vi "getControlMatrixDH.vi"(8 "error in (no error)":errorcluster, 11 "DataHandler in":refnum<class "DataHandler.lvclass">) -> (0 "error out":errorcluster, 1 "List of ColHads":string[](array[string]), 2 "ControlParameterArrayMatrix":string[][](array[string]), 3 "DataHandler out":refnum<class "DataHandler.lvclass">, 4 "Field Elements":string[](array[string]))   [LabVIEW 2017, in "DataHandler.lvclass"]
uses:
  DataHandler.lvclass
  DataHandler.lvclass/DataHandler.ctl
  <vilib>/drjdpowell/SQLite Library/SQL Connection/Execute SQL.vi
  <vilib>/drjdpowell/SQLite Library/SQLite.lvlib
  <vilib>/drjdpowell/SQLite Library/SQL Connection/Connection.lvclass
panel:
  in  "Control-Matrix":i32(listbox)=-1
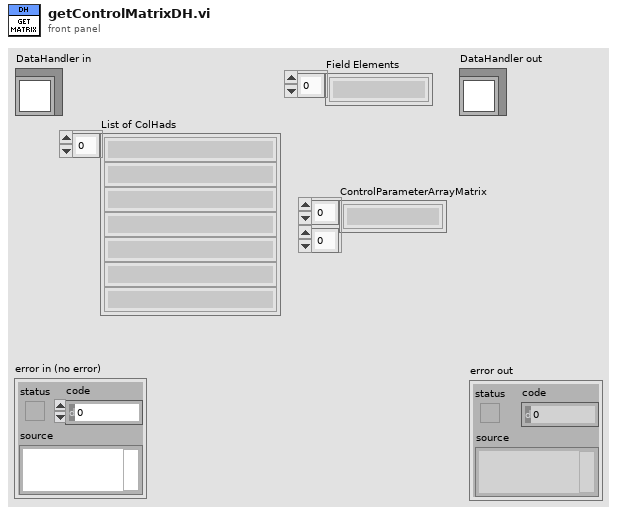
[diagram p1: front panel]
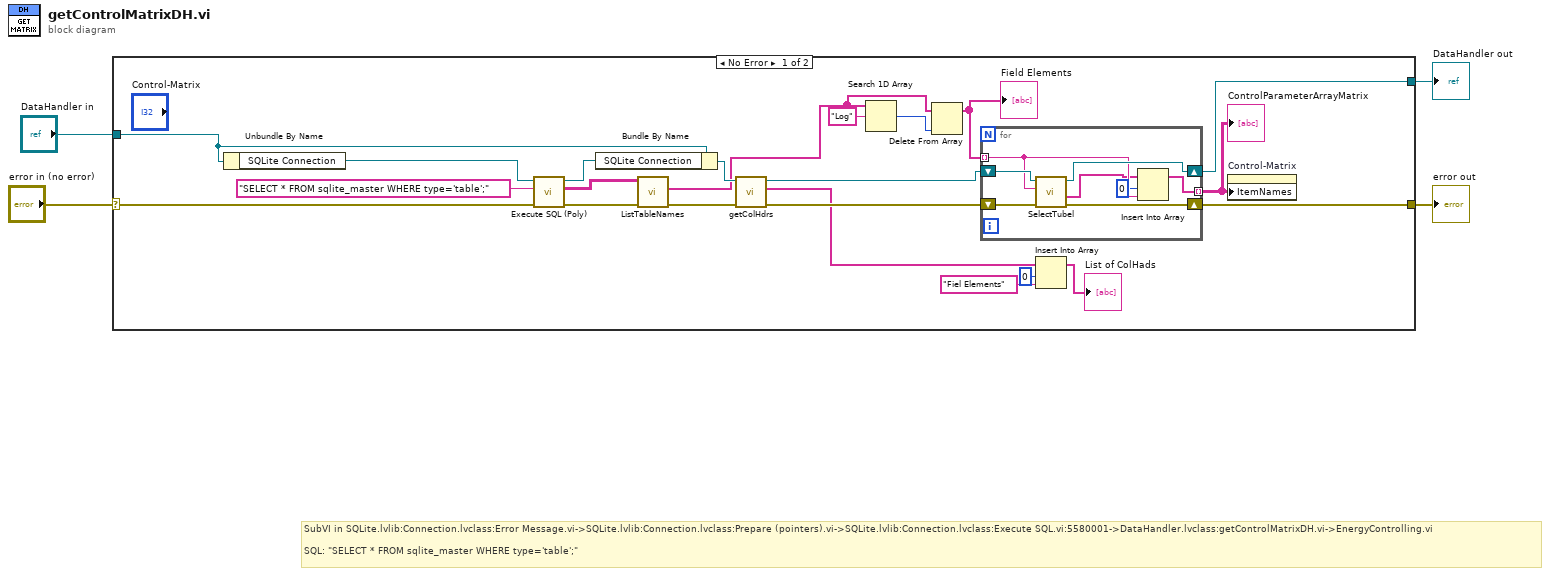
[diagram p0: block diagram]
diagram:
  # "SubVI in SQLite.lvlib:Connection.lvclass:Error Message.vi->SQLite.lvlib:Connection.lvclass:Prepare (pointers).vi->SQLite.lvlib:Connection.lvclass:Execute SQL.vi:5580001->DataHandler.lvclass:getControlMatrixDH.vi->EnergyControlling.vi\n\nSQL: \"SELECT * FROM sqlite_master WHERE type='table';\""
  n1 = case shown="No Error" "error in (no error)" {
    selector: "error in (no error)" -> [w19 w36]
    tunnel: [w25 w36] -> w3
    tunnel: [w24 w35] -> w1
    tunnel: "DataHandler in" -> [w18 w35]
    frame No Error {
      n2 = Unbundle By Name(w18) -> ("SQLite Connection"=w20:refnum<class "Connection.lvclass">)
      n3 = call-poly <vilib>:"Execute SQL (Poly).vi"("error in (no error)"=w19, "SQL"="SELECT * FROM sqlite_master WHERE type='table';" ("String"), "SQLite Connection in"=w20) -> ("error out"=w23:errorcluster, "Result Set"=w22:string[][], "SQLite Connection out"=w17:refnum<class "Connection.lvclass">)  [unwired: 5 in, 1 out]
      n4 = Bundle By Name(cluster=w18, "SQLite Connection"=w17) -> (w14:refnum<class "DataHandler.lvclass">)
      n5 = call "ListTableNames.vi"("error in (no error)"=w23, "Result Set"=w22) -> ("error out"=w16:errorcluster, "Table Names"=w6:string[])  [unwired: 7 in, 1 out]
      n6 = call-dynamic "getColHdrs.vi"("error in (no error)"=w16, "DataHandler in"=w14) -> ("error out"=w15:errorcluster, "List of ColHads"=w11:string[], "DataHandler out"=w13:refnum<class "DataHandler.lvclass">)  [unwired: 7 in]
      n7 = Search 1D Array(1D array=w6, element="Log") -> (index of element=w7:i32)  [unwired: 1 in]
      n8 = Delete From Array(array=w6, index=w7) -> (array with subset deleted=w5:string[])  [unwired: 1 in, 1 out]
      "Field Elements" <- w5
      n9 = for {
        shift-right: [w31] -> w24
        shift-left: w13 -> [w32]
        shift-right: [w33] -> w25
        shift-left: w15 -> [w34]
        tunnel: [w28] -> w26 mode=indexing
        tunnel: w5 -> [w30] mode=indexing
        n10 = call-dynamic "SelectTubel.vi"("error in (no error)"=w34, "Unique Object Identifier"=w30, "DataHandler in"=w32) -> ("error out"=w33:errorcluster, "ControlParameterArray"=w29:string[], "DataHandler out"=w31:refnum<class "DataHandler.lvclass">)  [unwired: 5 in, 1 out]
        n11 = Insert Into Array(array=w29, index=0, new element=w30) -> (w28:string[])
      }
      "ControlParameterArrayMatrix" <- w26
      n12 = Insert Into Array(array=w11, index=0, new element="Fiel Elements" ("new element/subarray")) -> (→"List of ColHads":string[])
      n13 = property on="Control-Matrix" class="MCListbox (strict)"("ItemNames"=w26) -> ()  [unwired: 2 in, 2 out]
    }
    frame Error {
    }
  }
  "error out" <- w3
  "DataHandler out" <- w1
